vi "2D Inverse Real FFT.vi"(10 "shift?":bool, 11 "FFT {X}":cdb[][](array[numeric])) -> (0 "error":i32, 3 "X":dbl[][](array[numeric]))   [LabVIEW 2020, in "NI_AALPro.lvlib"]
doc: "Computes the inverse discrete Fourier transform (IDFT) of the input sequence <B>FFT {X}</B>. You must manually select the polymorphic instance you want to use."
uses:
  NI_AALPro.lvlib
  <resource>/lvanlys.dll
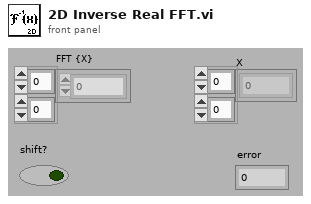
[diagram p1: front panel]
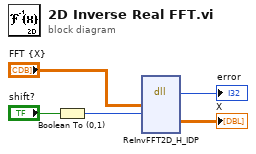
[diagram p0: block diagram]
diagram:
  n1 = Boolean To (0,1)(Boolean="shift?") -> (0, 1=w3:i16)
  n2 = dll-call lib="C:/Program Files (x86)/National Instruments/LabVIEW 2020/resource/lvanlys.*" fn="ReInvFFT2D_H_IDP"("xH"="FFT {X}", "shifted"=w3) -> ("return type"=→"error":i32, "yH"=→"X":dbl[][])  [unwired: 8 in, 2 out]
